vi "dfd_Maxflat Filter Design Extract Root.vi"(1 "input polynomial":dbl[](array[numeric])) -> (0 "extracted root":dbl)   [LabVIEW 2017, in "NI_DigFilter_Design.lvlib"]
doc: "Extracts the root of input polynomial, which has minimum distance with 0.5."
uses:
  <vilib>/addons/Digital Filter Design/NI_DigFilter_Design.lvlib
  <vilib>/Analysis/polynomials.llb/Polynomial Roots (DBL).vi
  <vilib>/Analysis/NI_AALPro.lvlib
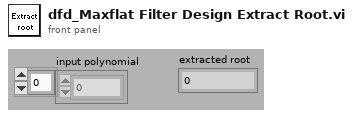
[diagram p1: front panel]
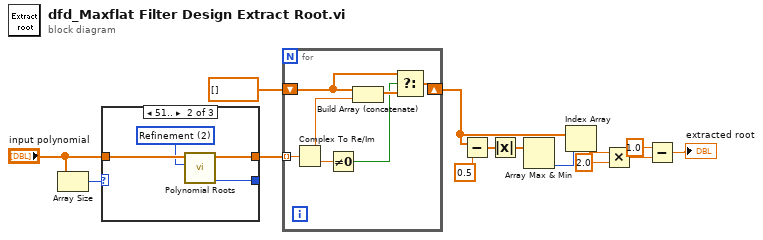
[diagram p0: block diagram]
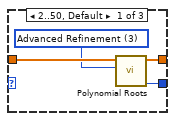
[diagram p2: hidden frame]
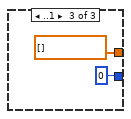
[diagram p3: hidden frame]
diagram:
  n1 = Array Size(array="input polynomial") -> (size(s)=w1:i32)
  n2 = case shown="51.." w1 {
    tunnel: [w18 w22 cdb[] [] ("Complex Pair Roots")] -> w3
    tunnel: "input polynomial" -> [w16 w20 _]
    tunnel: [w17 w21 0 ("error")] -> _
    frame 2..50, Default {
      w15 = u16 3 items=["General", "Simple Classification", "Refinement", "Advanced Refinement"] ("option")
      n3 = call-poly <vilib>:"Polynomial Roots.vi"("option"=w15, "P(x)"=w16) -> ("error"=w17:i32, "Roots"=w18:cdb[])  [unwired: 1 in, 7 out]
    }
    frame 51.. {
      w19 = u16 2 items=["General", "Simple Classification", "Refinement", "Advanced Refinement"] ("option")
      n4 = call-poly <vilib>:"Polynomial Roots.vi"("option"=w19, "P(x)"=w20) -> ("error"=w21:i32, "Roots"=w22:cdb[])  [unwired: 1 in, 7 out]
    }
    frame ..1 {
    }
  }
  n5 = for {
    tunnel: w3 -> [w31] mode=indexing
    shift-right: [w25] -> w4
    shift-left: dbl[] [] -> [w27]
    n6 = Complex To Re/Im(x + iy=w31) -> (x=w29:dbl, y=w30:dbl)
    n7 = Not Equal To 0?(x=w30) -> (x != 0?=w26:bool)
    n8 = Build Array (concatenate)(w27, w29) -> (w28:dbl[])
    n9 = Select(t=w27, s=w26, f=w28) -> (s? t:f=w25:dbl[])
  }
  n10 = Subtract(x=w4, y=0.5) -> (x-y=w7:dbl[])
  n11 = Absolute Value(x=w7) -> (abs(x)=w8:dbl[])
  n12 = Array Max & Min(array=w8) -> (min index (indices)=w9:i32)  [unwired: 3 out]
  n13 = Index Array(array=w4, index=w9) -> (element=w11:dbl)
  n14 = Multiply(x=w11, y=2.0) -> (x*y=w13:dbl)
  n15 = Subtract(x=1.0, y=w13) -> (x-y=→"extracted root":dbl)
